vi "32BitArray2ByteArray.vi"(11 "Array in":bool[](array[boolean])) -> (1 "Byte array out":u32[](array[numeric]))   [LabVIEW 2012]
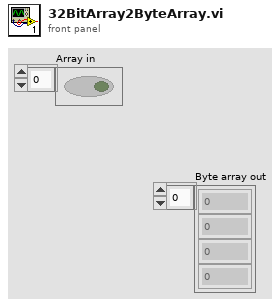
[diagram p1: front panel]
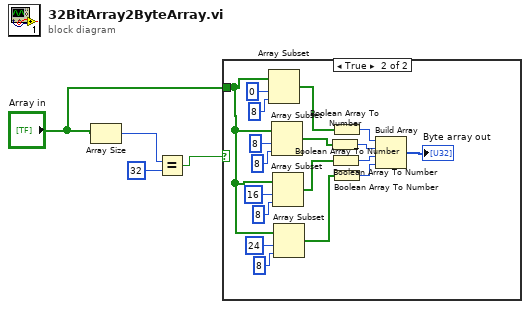
[diagram p0: block diagram]
diagram:
  n1 = Array Size(array="Array in") -> (size(s)=w1:i32)
  n2 = Equal?(x=w1, y=32) -> (x = y?=w3:bool)
  n3 = case shown="True" w3 {
    tunnel: "Array in" -> [_ w14]
    frame False {
    }
    frame True {
      n4 = Array Subset(array=w14, index=0, length=8) -> (w6:bool[])
      n5 = Array Subset(array=w14, index=8, length=8) -> (w7:bool[])
      n6 = Array Subset(array=w14, index=16, length=8) -> (w8:bool[])
      n7 = Array Subset(array=w14, index=24, length=8) -> (w9:bool[])
      n8 = Boolean Array To Number(Boolean array=w7) -> (number=w12:u32)
      n9 = Boolean Array To Number(Boolean array=w8) -> (number=w11:u32)
      n10 = Boolean Array To Number(Boolean array=w6) -> (number=w13:u32)
      n11 = Boolean Array To Number(Boolean array=w9) -> (number=w10:u32)
      n12 = Build Array(w13, w12, w11, w10) -> (→"Byte array out":u32[])
    }
  }
